vi "Read valve control.vi"(8 "error in (no error)":errorcluster, 10 "value":string, 11 "HT_in in":T1={"Z_HSw"=1, "Z_HSetState"=enum."on (closed)", "Reset_ALR"=FALSE}) -> (0 "error out":errorcluster, 2 "Data to Write":bool, 3 "HT1_in out":T1={"Z_HSw"=1, "Z_HSetState"=enum."initialization", "Reset_ALR"=FALSE})   [LabVIEW 2019, in "OPC addons.lvlib"]
uses:
  OPC addons.lvlib
  valves/ctl/Zr_control_VCH.ctl
  valves/ctl/Z_State_VCH.ctl
  <vilib>/JDP Science/JSONtext/String Subset.vi
  <vilib>/JDP Science/JSONtext/support/Strip Quotes and Unescape.vi
  <vilib>/JDP Science/JSONtext/support/Unescape JSON string.vi
  <vilib>/JDP Science/JSONtext/Parsing/Parse Full Path or Item Name.vi
  <vilib>/JDP Science/JSONtext/Offset/Find Item Locations by Path.vi
  <vilib>/JDP Science/JSONtext/JSONtext.lvlib
  valves/Valves.lvlib
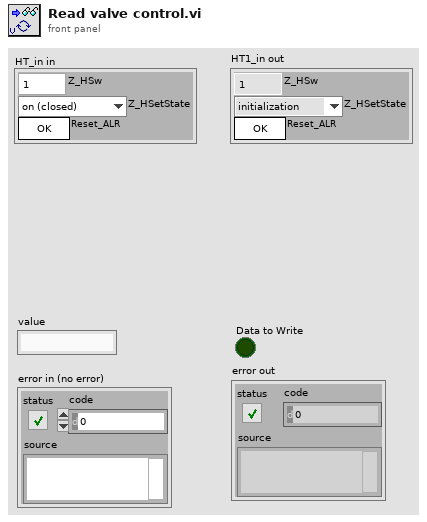
[diagram p1: front panel]
types:
  T1 = typedef "Valves.lvlib/Zr_control_VCH.ctl" = cluster{"Z_HSw":u8, "Z_HSetState":T2, "Reset_ALR":bool}
  T2 = typedef "Valves.lvlib/Z_State_VCH.ctl" = enum8{"initialization", "alarm", "disabled", "not ready", "closed ready", "reserv", "reserv1", "reserv2", "reserv3", "check", "on min", "open", "on (closed)"}
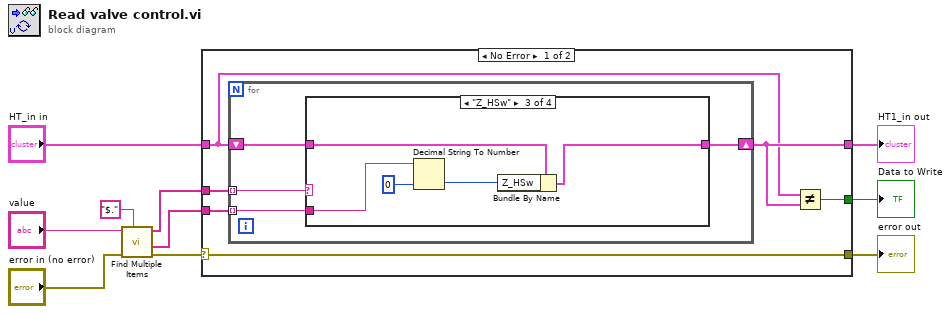
[diagram p0: block diagram]
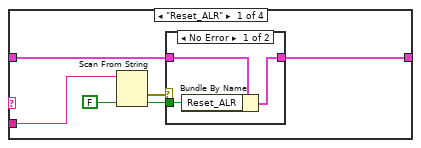
[diagram p2: hidden frame]
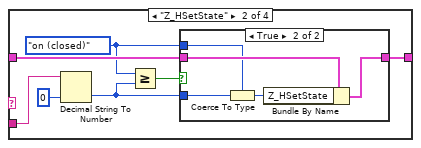
[diagram p4: hidden frame]
diagram:
  n1 = call <vilib>:"Find Multiple Items.vi"("$Path or Item Name"="$.", "error in (no error)"="error in (no error)", "JSON"="value") -> ("error out"=w7:errorcluster, "<JSON>"=w5:string[], "Item Names"=w10:string[])  [unwired: 5 in, 1 out]
  n2 = case shown="No Error" w7 {
    selector: w7 -> [w13 w50]
    tunnel: w10 -> [w16 _]
    tunnel: "HT_in in" -> [w11 w51]
    tunnel: w5 -> [w15 _]
    tunnel: [w12 w51] -> w6
    tunnel: [w14 _] -> w2
    tunnel: [w13 w50] -> w1
    frame No Error {
      n3 = for {
        shift-right: [w18] -> w12
        shift-left: w11 -> [w20]
        tunnel: w16 -> [w17] mode=indexing
        tunnel: w15 -> [w19] mode=indexing
        n4 = case shown="\"Z_HSw\"" w17 {
          tunnel: w20 -> [w26 w37 w48 w49]
          tunnel: w19 -> [w23 w35 w45 _]
          tunnel: [w25 w34 w44 w49] -> w18
          frame "Reset_ALR" {
            n5 = Scan From String(input string=w23, default 1=FALSE ("use system decimal point (T)")) -> (error out=w21:errorcluster, output 1=w22:bool)  [unwired: 3 in, 2 out]
            n6 = case shown="No Error" w21 {
              tunnel: w26 -> [w29 w30]
              tunnel: [w28 w30] -> w25
              tunnel: w22 -> [w27 _]
              frame No Error {
                n7 = Bundle By Name(cluster=w29, "Reset_ALR"=w27) -> (w28:T1)
              }
              frame Error {
              }
            }
          }
          frame "Z_HSetState" {
            w31 = Z_State_VCH."on (closed)" ("Y_HSetState")
            n8 = Decimal String To Number(string=w35, default (0L)=u8 0 ("Z_HSw")) -> (number=w32:u8)  [unwired: 1 in, 1 out]
            n9 = Greater Or Equal?(x=w31, y=w32) -> (x >= y?=w33:bool)
            n10 = case shown="True" w33 {
              tunnel: w37 -> [w38 w43]
              tunnel: [w38 w42] -> w34
              tunnel: w31 -> [_ w40]
              tunnel: w32 -> [_ w39]
              frame False {
              }
              frame True {
                n11 = Coerce To Type(0:w39, 1:w40) -> (2:w41:T2)
                n12 = Bundle By Name(cluster=w43, "Z_HSetState"=w41) -> (w42:T1)
              }
            }
          }
          frame "Z_HSw" {
            n13 = Decimal String To Number(string=w45, default (0L)=u32 0 ("Z_HSw")) -> (number=w46:u32)  [unwired: 1 in, 1 out]
            n14 = Bundle By Name(cluster=w48, "Z_HSw"=w46) -> (w44:T1)
          }
          frame Default {
          }
        }
      }
      n15 = Not Equal?(x=w11, y=w12) -> (x != y?=w14:bool)
    }
    frame Error {
    }
  }
  "HT1_in out" <- w6
  "Data to Write" <- w2
  "error out" <- w1
